vi "题目 5.vi"() -> ()   [LabVIEW 2017]
panel:
  out "油量指示灯":bool
  out "时间":dbl
  in  "停止":bool
  in  "控制面板":T1 {"档位" scale=0.0..6.0; "油门" scale=0.0..10.0}
  out "显示面板":T2 {"油量" scale=0.0..200.0; "速度（km/h）" scale=0.0..300.0; "转速（r/s）" scale=0.0..8000.0}
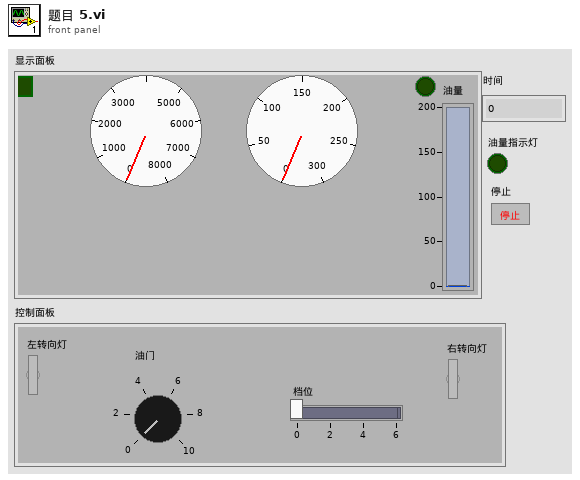
[diagram p1: front panel]
types:
  T1 = cluster{"左转向灯":bool, "右转向灯":bool, "油门":dbl, "档位":dbl}
  T2 = cluster{"左转向灯":bool, "右转向灯 2":bool, "转速（r/s）":dbl, "速度（km/h）":dbl, "油量":dbl}
  T3 = cluster{"左转向灯":bool, "右转向灯":bool, dbl, dbl, "real":dbl}
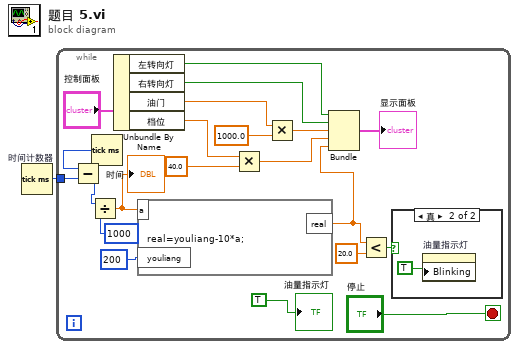
[diagram p0: block diagram]
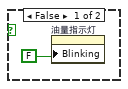
[diagram p2: hidden frame]
diagram:
  n1 = Tick Count (ms) "时间计数器"() -> (millisecond timer value=w1:u32)
  n2 = while {
    tunnel: w1 -> [w9]
    stop <- "停止" stop-if-true
    n3 = Tick Count (ms)() -> (millisecond timer value=w13:u32)
    n4 = Subtract(x=w13, y=w9) -> (x-y=w15:u32)
    n5 = Divide(x=w15, y=1000) -> (x/y=w14:dbl)
    "时间" <- w14
    n6 = Unbundle By Name("控制面板") -> ("左转向灯"=w6:bool, "右转向灯"=w7:bool, "油门"=w8:dbl, "档位"=w20:dbl)
    n7 = formula code="real=youliang-10*a;"("a"=w14, "youliang"=200) -> ("real"=w3:dbl)
    n8 = Multiply(x=w20, y=40.0) -> (x*y=w5:dbl)
    n9 = Multiply(x=w8, y=1000.0) -> (x*y=w18:dbl)
    n10 = Bundle("左转向灯"=w6, "右转向灯"=w7, w18, w5, "real"=w3) -> (→"显示面板":T3)  [unwired: 1 in]
    n11 = Less?(x=w3, y=20.0) -> (x < y?=w16:bool)
    n12 = case shown="真" w16 {
      frame False {
        n13 = property on="油量指示灯" class="Bool (严格)"("Blinking"=FALSE) -> ()  [unwired: 2 in, 2 out]
      }
      frame True {
        n14 = property on="油量指示灯" class="Bool (严格)"("Blinking"=TRUE) -> ()  [unwired: 2 in, 2 out]
      }
    }
    "油量指示灯" <- TRUE
  }
